vi "VOT_Reflect&Unifority.vi"(9 "file (use dialog)":path=path "C:/Users/user/Desktop/5FKHB7A6/test_report.txt") -> (0 "Unifority":string[](array[string]), 1 "Reflect":string, 2 "Result":bool)   [LabVIEW 2017]
panel:
  out "Array":string[][](array[string])
  # "[Internal Reflection]\nDeviation          : 29.279353017271404\nResult             : FAIL\n\n\n[Uniformity]\nInitial brightness : 3.5%\nMean uniformity    : 241.6367\nDeviation          : 29.279353017271404\nAdjusted brightness: 4.0%\nMean uniformity    : 240.6367\nDeviation          : 28.279353017271404\nResult             : FAIL"
  # "78.03311169779147"
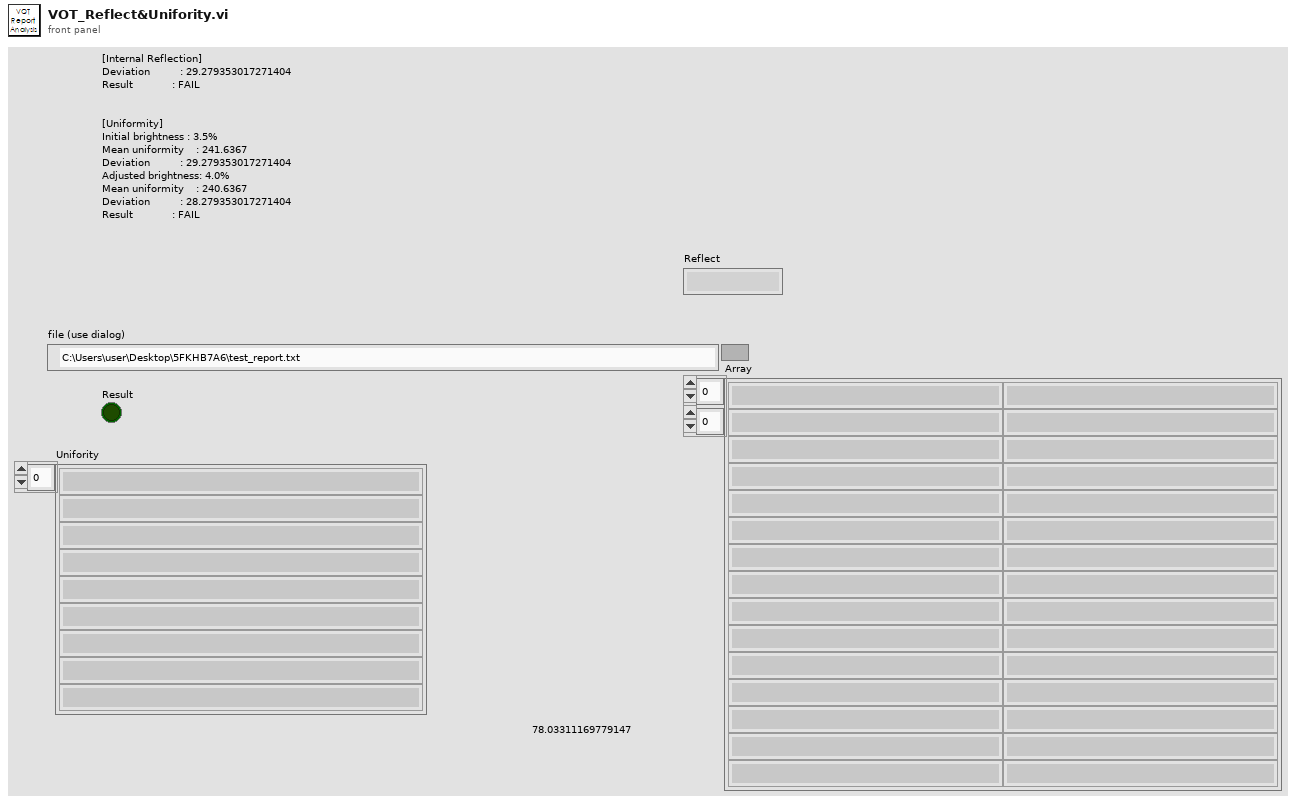
[diagram p1: front panel]
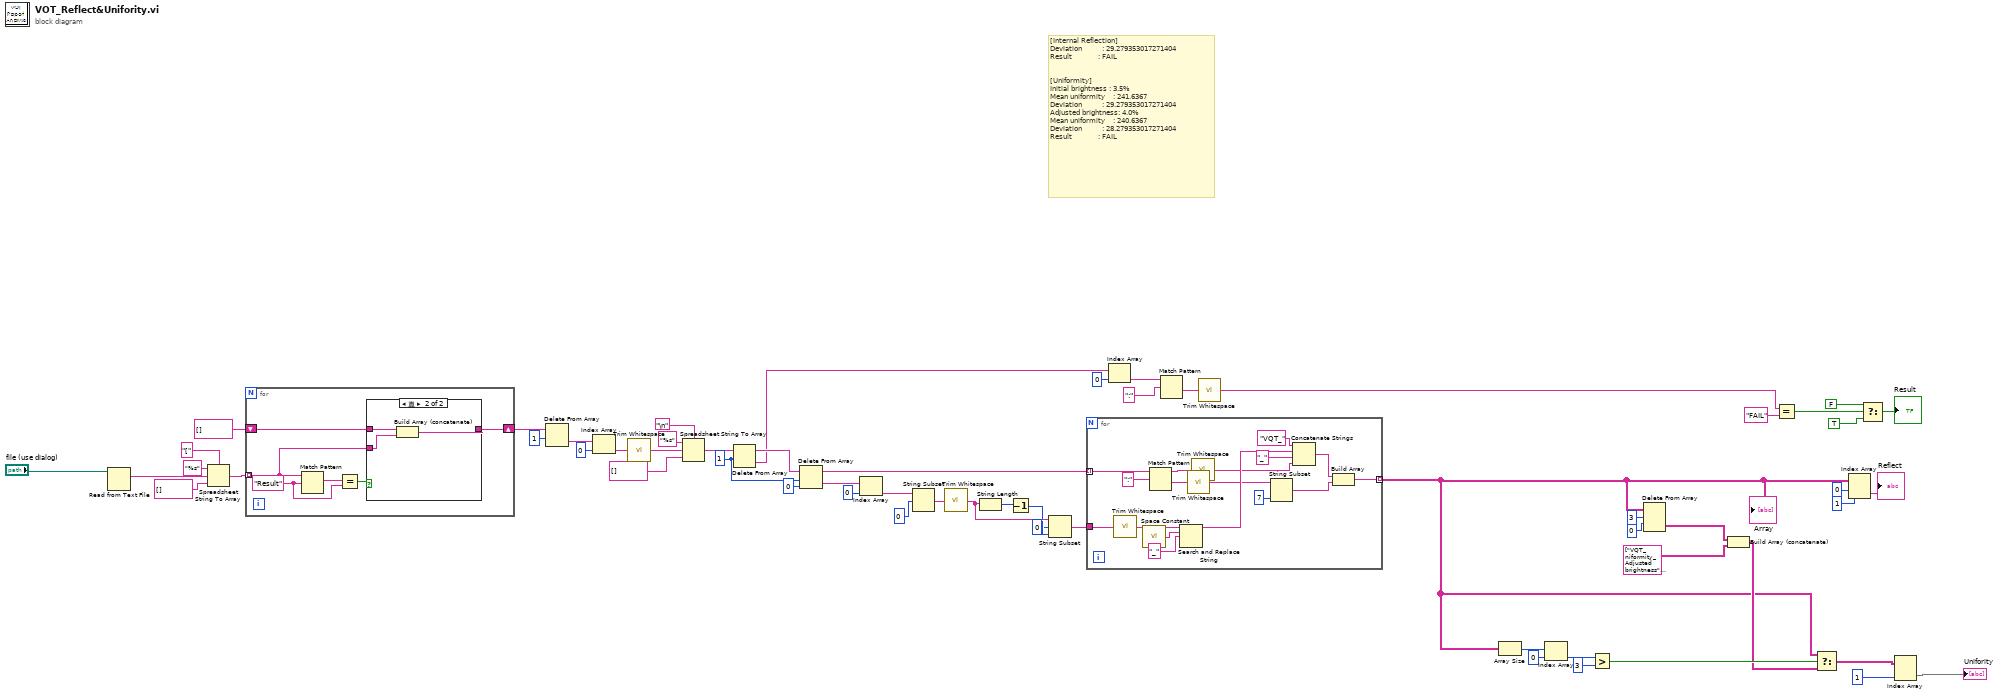
[diagram p0: block diagram]
diagram:
  w52 = 1 ("length")
  # "[Internal Reflection]\nDeviation          : 29.279353017271404\nResult             : FAIL\n\n\n[Uniformity]\nInitial brightness : 3.5%\nMean uniformity    : 241.6367\nDeviation          : 29.279353017271404\nAdjusted brightness: 4.0%\nMean uniformity    : 240.6367\nDeviation          : 28.279353017271404\nResult             : FAIL"
  n1 = Read from Text File(file (use dialog)="file (use dialog)") -> (text=w30:string)  [unwired: 3 in, 3 out]
  n2 = Spreadsheet String To Array(delimiter (Tab)="[", format string="%s", spreadsheet string=w30, array type (2D Dbl)=string[] []) -> (array=w31:string[])
  n3 = for {
    shift-right: [w60] -> w29
    shift-left: string[] [] -> [w62]
    tunnel: w31 -> [w61] mode=indexing
    w64 = "Result" ("regular expression")
    n4 = Match Pattern(string=w61, regular expression=w64) -> (match substring=w65:string)  [unwired: 1 in, 3 out]
    n5 = Equal?(x=w65, y=w64) -> (x = y?=w63:bool)
    n6 = case shown="真" w63 {
      tunnel: w62 -> [w66 w69]
      tunnel: w61 -> [_ w68]
      tunnel: [w66 w67] -> w60
      frame False {
      }
      frame True {
        n7 = Build Array (concatenate)(w69, w68) -> (w67:string[])
      }
    }
  }
  n8 = Delete From Array(array=w29, length=1) -> (deleted portion=w27:string[])  [unwired: 1 in, 1 out]
  n9 = Index Array(array=w27, index=0) -> (element=w26:string)
  n10 = call <vilib>:"Trim Whitespace.vi"("string"=w26) -> ("trimmed string"=w58:string)  [unwired: 1 in]
  n11 = Spreadsheet String To Array(delimiter (Tab)="\n", format string="%s", spreadsheet string=w58, array type (2D Dbl)=string[] []) -> (array=w54:string[])
  n12 = Delete From Array(array=w54, length=w52) -> (deleted portion=w50:string[], array with subset deleted=w53:string[])  [unwired: 1 in]
  n13 = Delete From Array(array=w53, length=w52, index=0) -> (deleted portion=w43:string[], array with subset deleted=w45:string[])
  n14 = Index Array(array=w43, index=0) -> (element=w42:string)
  n15 = String Subset(string=w42, offset (0)=0) -> (substring=w40:string)  [unwired: 1 in]
  n16 = call <vilib>:"Trim Whitespace.vi"("string"=w40) -> ("trimmed string"=w38:string)  [unwired: 1 in]
  n17 = String Length(string=w38) -> (length=w39:i32)
  n18 = Decrement(x=w39) -> (x-1=w37:i32)
  n19 = String Subset(string=w38, offset (0)=0, length (rest)=w37) -> (substring=w36:string)
  n20 = for {
    tunnel: w45 -> [w84] mode=indexing
    tunnel: w36 -> [w83]
    tunnel: [w79] -> w1 mode=indexing
    n21 = call <vilib>:"Trim Whitespace.vi"("string"=w83) -> ("trimmed string"=w82:string)  [unwired: 1 in]
    n22 = call <vilib>:"Space Constant.vi"() -> ("String"=w81:string)
    n23 = Match Pattern(string=w84, regular expression=":") -> (before substring=w78:string, after substring=w86:string)  [unwired: 1 in, 2 out]
    n24 = Search and Replace String(input string=w82, search string=w81, replace string="_") -> (result string=w75:string)  [unwired: 5 in, 3 out]
    n25 = call <vilib>:"Trim Whitespace.vi"("string"=w86) -> ("trimmed string"=w72:string)  [unwired: 1 in]
    n26 = call <vilib>:"Trim Whitespace.vi"("string"=w78) -> ("trimmed string"=w74:string)  [unwired: 1 in]
    n27 = String Subset(string=w72, length (rest)=7 ("length (rest)")) -> (substring=w70:string)  [unwired: 1 in]
    n28 = Concatenate Strings("VQT_" ("string"), w75, "_" ("string"), w74) -> (w73:string)
    n29 = Build Array(w73, w70) -> (w79:string[])
  }
  "Array" <- w1
  n30 = Index Array(array=w50, index=0) -> (element=w48:string)
  n31 = Match Pattern(string=w48, regular expression=":") -> (after substring=w46:string)  [unwired: 1 in, 3 out]
  n32 = call <vilib>:"Trim Whitespace.vi"("string"=w46) -> ("trimmed string"=w14:string)  [unwired: 1 in]
  n33 = Array Size(array=w1) -> (size(s)=w24:i32[])
  n34 = Index Array(array=w24, index=0) -> (element=w22:i32)
  n35 = Greater?(x=w22, y=3) -> (0:w16:bool)
  n36 = Delete From Array(array=w1, length=3, index (row)=0) -> (deleted portion=w18:string[][])  [unwired: 1 in, 1 out]
  n37 = Build Array (concatenate)(w18, string[][] [["VQT_niformity_Adjusted brightness", "NA"], ["VQT_niformity_Mean uniformity", "NA"], ["VQT_niformity_Deviation", "NA"]] ("Adjusted")) -> (w15:string[][])
  n38 = Equal?(x=w14, y="FAIL") -> (x = y?=w12:bool)
  n39 = Select(t=w1, s=w16, f=w15) -> (s? t:f=w3:string[][])
  n40 = Index Array(array=w1, index (row)=0, index (col)=1 ("disabled index (col)")) -> (element=→"Reflect":string)
  n41 = Select(t=FALSE, s=w12, f=TRUE) -> (s? t:f=→"Result":bool)
  n42 = Index Array(array=w3, index (col)=1 ("disabled index (col)")) -> (element=→"Unifority":string[])  [unwired: 1 in]
